vi "VI Tree.vi"   [LabVIEW 2017, in "Samwontech TEMP2xxx.lvlib"]
doc: "This is the instrument driver for the <INSTRUMENT NAME>. The VI Tree displays all the user-callable VIs of the instrument driver in an organized table."
uses:
  <instrlib>/Samwontech TEMP2xxx/Samwontech TEMP2xxx.lvlib
panel:
  # "(c) 2014 <Enter Company Name Here>.  ALL RIGHTS RESERVED."
  # "SEE DIAGRAM\nFOR VI TREE."
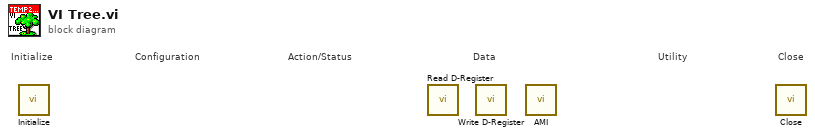
[diagram p0: block diagram]
diagram:
  # "Configuration"
  # "Utility"
  # "Data"
  # "Action/Status"
  # "Close"
  # "Initialize"
  n1 = call <instrlib>:"Initialize.vi"() -> ()  [unwired: 10 in, 2 out]
  n2 = call <instrlib>:"Read D-Register.vi"() -> ()  [unwired: 8 in, 4 out]
  n3 = call <instrlib>:"Write D-Register.vi"() -> ()  [unwired: 9 in, 3 out]
  n4 = call <instrlib>:"AMI.vi"() -> ()  [unwired: 11 in, 5 out]
  n5 = call <instrlib>:"Close.vi"() -> ()  [unwired: 11 in, 1 out]
